vi "T7 Stream Select Tasks KAG.vi"(7 "Task Selector Array":string[](array[combo]), 8 "error in":errorcluster, 9 "Secondary Stream Configurations":T3={"Settling Delay (*5 us)"=0.0, "Clock Source"=0, "Auto Target"=1} {"Auto Target" max=5000 step=1; "Clock Source" max=2 step=2; "Settling Delay (*5 us)" max=255 step=1}, 10 "Strm Config in":T1={"Scan Rate (Hz)"=1000.0, "Samples Per Packet"=512, "Resolution Index"=0, "Buffer Size (bytes)"=32768, "NumScans"=1500, "Read Timeout (ms)"=5000, "Scan Table"=[{"Channel"=0, "BipGain"=0, "Input Config"="Single-Ended"}, {"Channel"=1, "BipGain"=0, "Input Config"="Single-Ended"}, {"Channel"=2, "BipGain"=0, "Input Config"="Single-Ended"}, {"Channel"=3, "BipGain"=0, "Input Config"="Single-Ended"}]} {"Samples Per Packet" max=512 step=1; "Buffer Size (bytes)" max=32768 step=1; "Resolution Index" max=8 step=1; "Scan Rate (Hz)" max=100000; "Scan Table"."BipGain" items=["x1", "x10", "x100", "x1000"]; "Scan Table"."Channel" step=1}, 11 "IP Config in":T4={"Connection ID In"=refnum, "Connection ID Out"=refnum, "Device IP"="192.168.126.147", "Port"=502}) -> (0 "error out":errorcluster, 2 "Strm Config out":T1={"Scan Rate (Hz)"=1000.0, "Samples Per Packet"=512, "Resolution Index"=0, "Buffer Size (bytes)"=32768, "NumScans"=1500, "Read Timeout (ms)"=5000, "Scan Table"=[{"Channel"=0, "BipGain"=0, "Input Config"="Single-Ended"}, {"Channel"=1, "BipGain"=0, "Input Config"="Single-Ended"}, {"Channel"=2, "BipGain"=0, "Input Config"="Single-Ended"}, {"Channel"=3, "BipGain"=0, "Input Config"="Single-Ended"}]} {"Samples Per Packet" max=512 step=1; "Buffer Size (bytes)" max=32768 step=1; "Resolution Index" max=8 step=1; "Scan Rate (Hz)" max=100000; "Scan Table"."BipGain" items=["x1", "x10", "x100", "x1000"]; "Scan Table"."Channel" step=1}, 3 "IP Config out":T2={"Connection ID In"=refnum, "Connection ID Out"=refnum, "Device IP"="", "Port"=502})   [LabVIEW 2015]
uses:
  T7 Stream Config KAG.ctl
  T7 IP Config KAG.ctl
  T7 Secondary Configs KAG.ctl
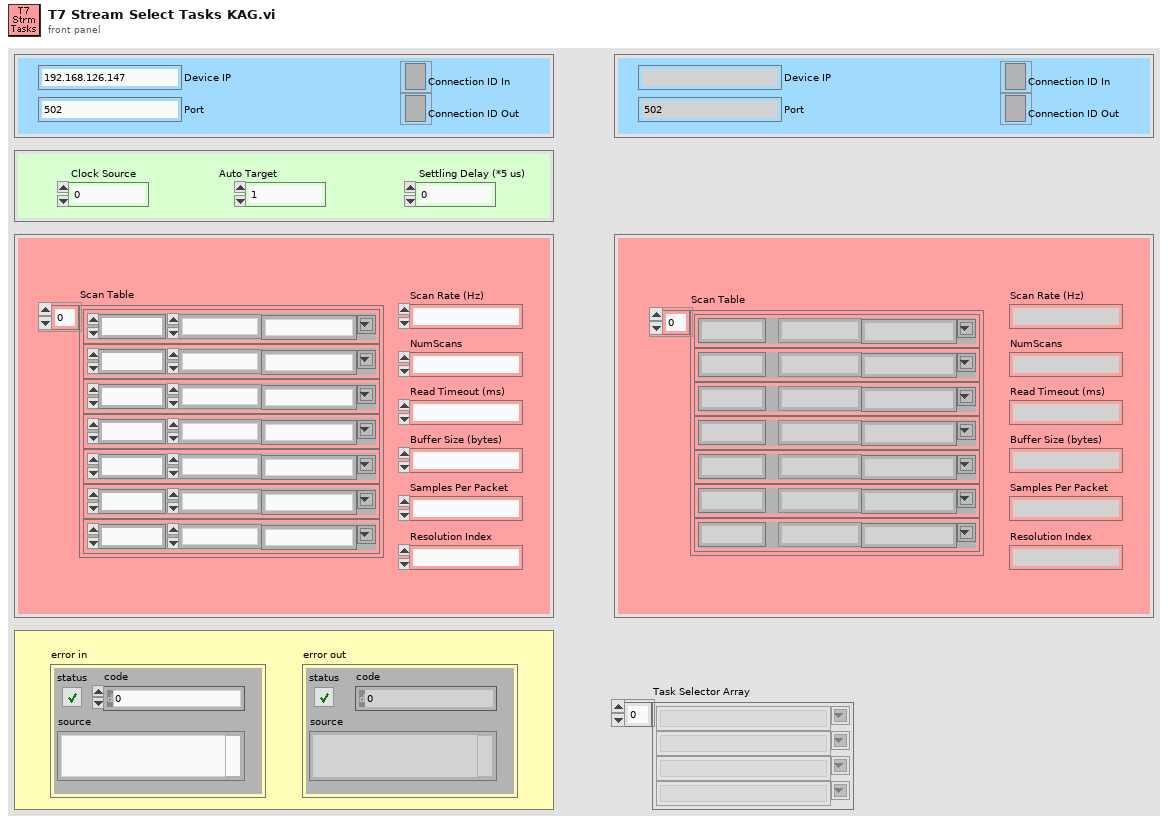
[diagram p1: front panel]
types:
  T1 = typedef "T7 Stream Config KAG.ctl" = cluster{"Scan Rate (Hz)":sgl, "Samples Per Packet":u32, "Resolution Index":u32, "Buffer Size (bytes)":u32, "NumScans":u32, "Read Timeout (ms)":u32, "Scan Table":cluster{"Channel":u32, "BipGain":u32, "Input Config":string}[]}
  T2 = cluster{"Connection ID In":refnum<k5>, "Connection ID Out":refnum<k5>, "Device IP":string, "Port":i32}
  T3 = typedef "T7 Secondary Configs KAG.ctl" = cluster{"Settling Delay (*5 us)":sgl, "Clock Source":u32, "Auto Target":u32}
  T4 = typedef "T7 IP Config KAG.ctl" = cluster{"Connection ID In":refnum<k5>, "Connection ID Out":refnum<k5>, "Device IP":string, "Port":i32}
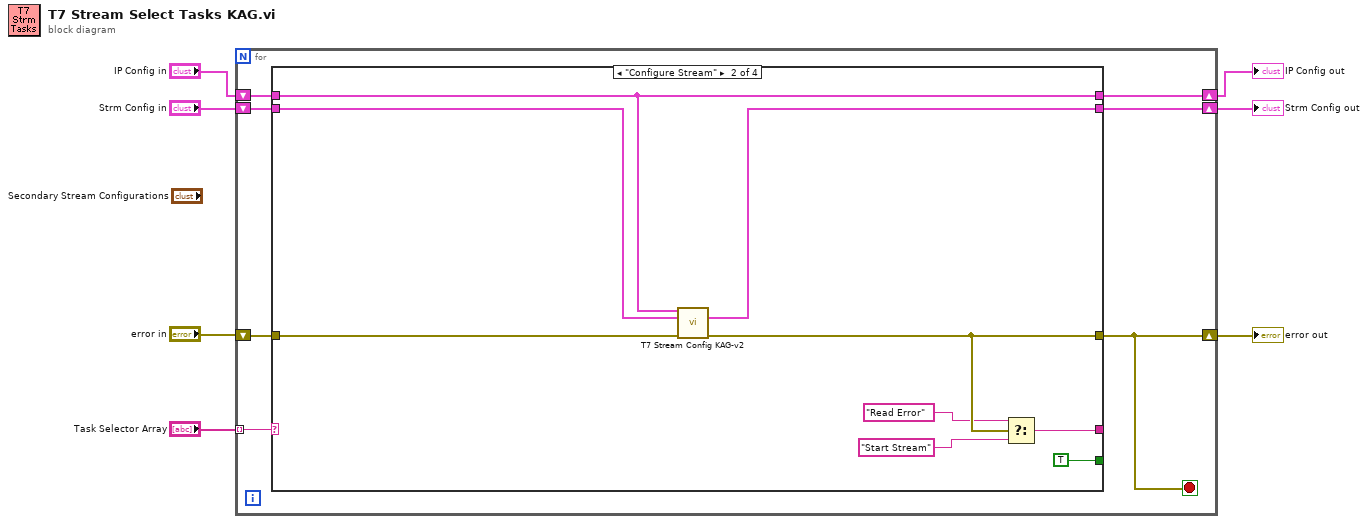
[diagram p0: block diagram]
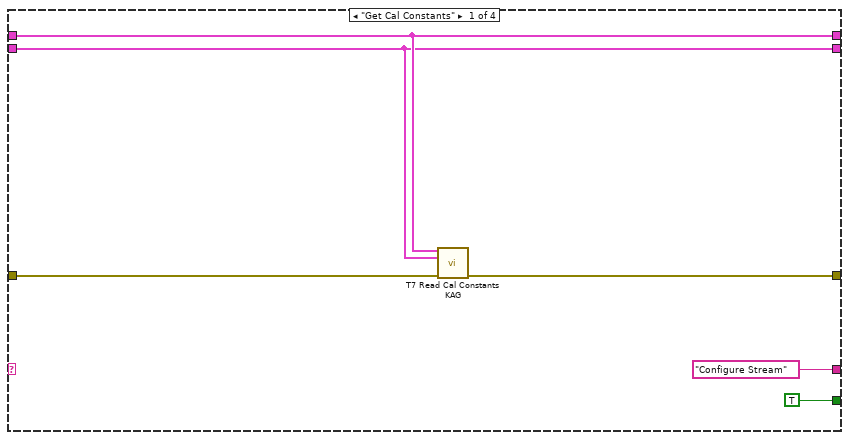
[diagram p2: hidden frame]
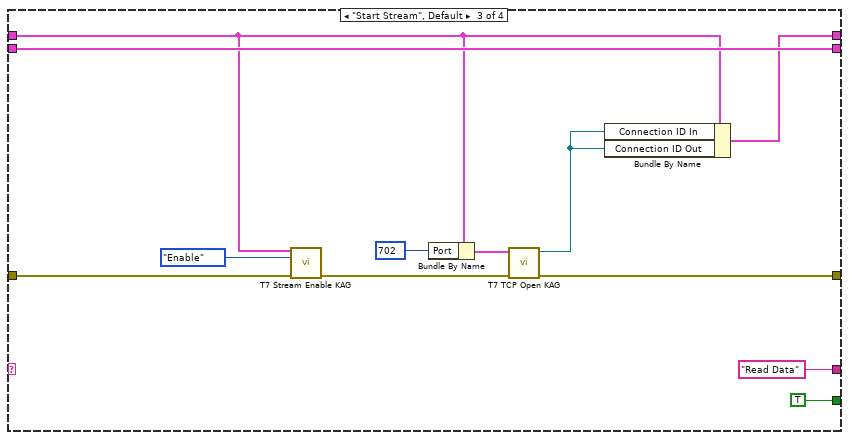
[diagram p3: hidden frame]
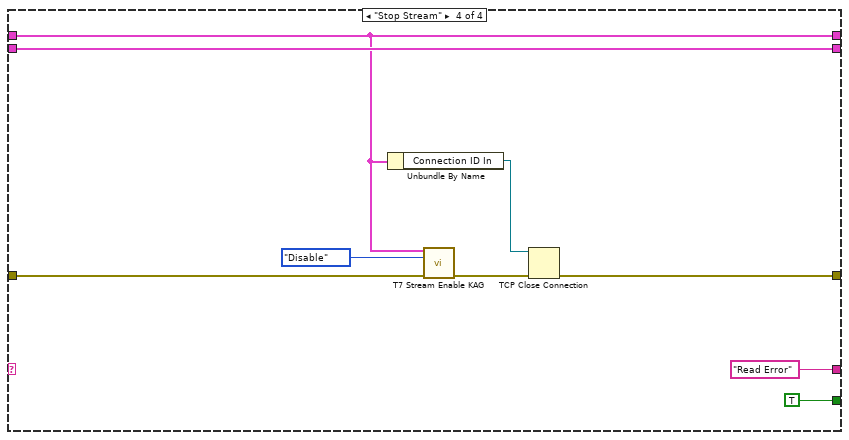
[diagram p4: hidden frame]
diagram:
  n1 = for {
    shift-right: [w9] -> w2
    shift-left: "error in" -> [w14]
    shift-right: [w13] -> w4
    shift-left: "IP Config in" -> [w12]
    shift-right: [w11] -> w5
    shift-left: "Strm Config in" -> [w10]
    tunnel: "Task Selector Array" -> [w8] mode=indexing
    stop <- w9 stop-if-true
    n2 = case shown="\"Configure Stream\"" w8 {
      tunnel: [TRUE TRUE TRUE TRUE] -> _
      tunnel: ["Configure Stream" ("f") w24 "Read Data" "Read Error"] -> _
      tunnel: [w19 w27 w37 w48] -> w9
      tunnel: w14 -> [w20 w22 w39 w46]
      tunnel: [w16 w28 w31 w43] -> w13
      tunnel: w12 -> [w16 w28 w32 w43]
      tunnel: [w15 w23 w34 w47] -> w11
      tunnel: w10 -> [w15 w21 w34 w47]
      frame "Get Cal Constants" {
        n3 = call "T7 Read Cal Constants KAG.vi"("IP Configuration"=w16, "Stream Configuration"=w15, "error in"=w20) -> ("error out"=w19:errorcluster)  [unwired: 11 in, 1 out]
      }
      frame "Configure Stream" {
        n4 = call "T7 Stream Config KAG-v2.vi"("IP Configuration"=w28, "Stream Configuration"=w21, "error in"=w22) -> ("Strm Config Out"=w23:T1, "error out"=w27:errorcluster)  [unwired: 11 in]
        n5 = Select(t="Read Error", s=w27, f="Start Stream") -> (s? t:f=w24:string)
      }
      frame "Start Stream", Default {
        n6 = call "T7 Stream Enable KAG.vi"("IP Configuration"=w32, "Enable"=enum32{"Disable", "Enable"}."Enable", "error in"=w39) -> ("error out"=w38:errorcluster)  [unwired: 12 in]
        n7 = Bundle By Name(cluster=w32, "Port"=702) -> (w35:T4)
        n8 = call "T7 TCP Open KAG.vi"("error in"=w38, "IP Configuration"=w35) -> ("error out"=w37:errorcluster, "connection ID out"=w30:refnum<k5>)  [unwired: 8 in]
        n9 = Bundle By Name(cluster=w32, "Connection ID In"=w30, "Connection ID Out"=w30) -> (w31:T4)
      }
      frame "Stop Stream" {
        n10 = Unbundle By Name(w43) -> ("Connection ID In"=w42:refnum<k5>)
        n11 = call "T7 Stream Enable KAG.vi"("IP Configuration"=w43, "Enable"=enum32{"Disable", "Enable"}."Disable", "error in"=w46) -> ("error out"=w45:errorcluster)  [unwired: 12 in]
        n12 = TCP Close Connection(connection ID=w42, error in (no error)=w45) -> (error out=w48:errorcluster)  [unwired: 1 in, 1 out]
      }
    }
  }
  "error out" <- w2
  "IP Config out" <- w4
  "Strm Config out" <- w5
